vi "FindSubpanels.Config.vi"(6 "Append (F)":bool, 8 "error in":errorcluster, 9 "Ini Cluster Name":string, 10 "Path":path, 11 "SMO.UI.MAUI in":refnum<class "SMO.UI.MAUI.lvclass">) -> (0 "error out":errorcluster, 3 "SMO.UI.MAUI out":refnum<class "SMO.UI.MAUI.lvclass">)   [LabVIEW 2020, in "SMO.UI.MAUI.lvclass"]
doc: "Load subpanels from a configuration file. Ini cluster name is optional, and a blank input will search for a cluster with a name of \"Subpanels\". The cluster must contain a single element of type array of paths. Append is to tell Maui that you want to add these to a list that already exists, rather than overwrite an existing list."
uses:
  SMO.UI.MAUI.lvclass
  <vilib>/Utility/config.llb/NI_LVConfig.lvlib
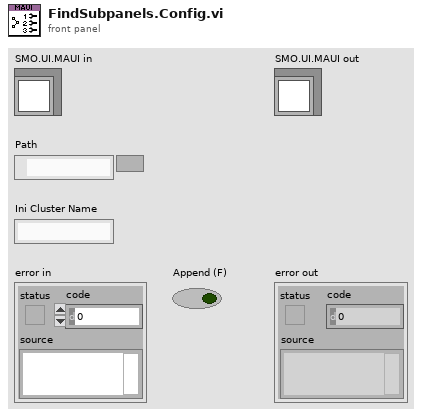
[diagram p1: front panel]
types:
  T1 = typedef "NI_LVConfig.lvlib/Config Data RefNum.ctl" = refnum<k1>
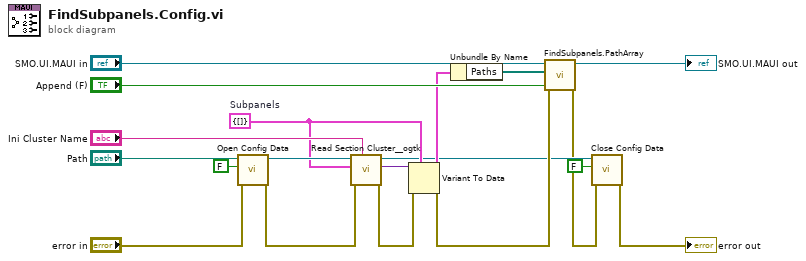
[diagram p0: block diagram]
diagram:
  w9 = cluster{"Paths":path[]} {"Paths"=[]}  # Subpanels
  n1 = call <vilib>:"Open Config Data.vi"("error in (no error)"="error in", "create file if necessary (T)"=FALSE, "configuration file path"="Path") -> ("error out"=w12:errorcluster, "refnum"=w16:T1)  [unwired: 6 in, 1 out]
  n2 = call <userlib>:"Read Section Cluster__ogtk.vi"("section (optional)"="Ini Cluster Name", "error in (no error)"=w12, "Section Formatted Cluster Type"=w9, "refnum"=w16) -> ("error out"=w10:errorcluster, "Section Formatted Cluster"=w11:variant, "dup refnum"=w5:T1)  [unwired: 3 in, 2 out]
  n3 = Variant To Data(error in=w10, type=w9, Variant=w11) -> (data=w8:cluster{"Paths":path[]}, error out=w6:errorcluster)
  n4 = Unbundle By Name(w8) -> ("Paths"=w7:path[])
  n5 = call-dynamic "FindSubpanels.PathArray.vi"("Append (F)"="Append (F)", "error in"=w6, "Subpanel List"=w7, "SMO.UI.MAUI in"="SMO.UI.MAUI in") -> ("error out"=w3:errorcluster, "SMO.UI.MAUI out"=→"SMO.UI.MAUI out":refnum<class "SMO.UI.MAUI.lvclass">)  [unwired: 6 in]
  n6 = call <vilib>:"Close Config Data.vi"("error in (no error)"=w3, "write file if changed (T)"=FALSE, "refnum"=w5) -> ("error out"=→"error out":errorcluster)  [unwired: 7 in, 1 out]
